vi "Number_Display_Subvi.vi"(6 "Str_x1":refnum<vi>, 7 "Totol Number":i32, 8 "Str_10":refnum<vi>, 9 "Str_x100":refnum<vi>, 10 "Str_x1000":refnum<vi>, 11 "Str_x10000":refnum<vi>) -> ()   [LabVIEW 2013]
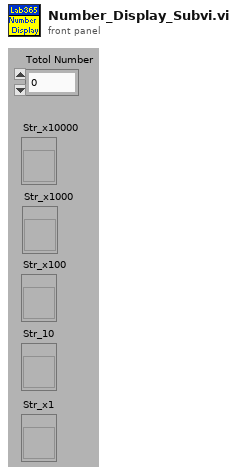
[diagram p1: front panel]
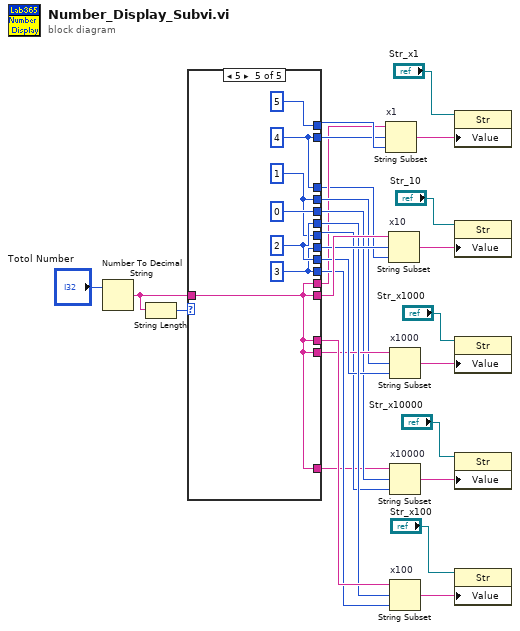
[diagram p0: block diagram]
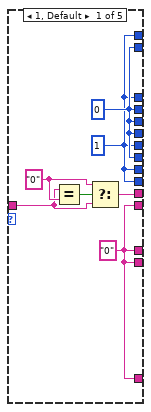
[diagram p2: hidden frame]
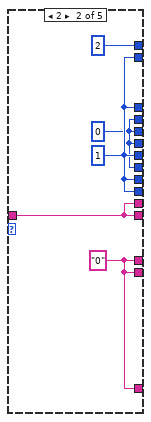
[diagram p3: hidden frame]
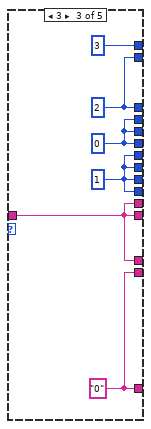
[diagram p4: hidden frame]
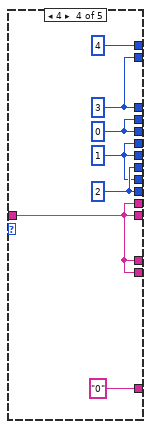
[diagram p5: hidden frame]
diagram:
  n1 = Number To Decimal String(number="Totol Number") -> (decimal integer string=w24:string)  [unwired: 1 out]
  n2 = String Length(string=w24) -> (length=w25:i32)
  n3 = case shown="5" w25 {
    tunnel: w24 -> [w31 w37 w45 w52 w60]
    tunnel: [w32 w37 w45 w52 w60] -> w11
    tunnel: [w30 w38 w41 w47 0 ("长度（剩余）")] -> w14
    tunnel: [w30 w39 w43 w50 w54] -> w16
    tunnel: [w35 w37 w45 w52 w60] -> w23
    tunnel: [w30 w38 w42 w49 w55] -> w22
    tunnel: [w29 w39 w43 w50 w54] -> w9
    tunnel: [w35 w36 w45 w52 w60] -> w21
    tunnel: [w30 w38 w41 w48 w58] -> w20
    tunnel: [w29 w39 w42 w49 w55] -> w19
    tunnel: [w35 w36 w44 w52 w60] -> w15
    tunnel: [w30 w38 w41 w47 w56] -> w13
    tunnel: [w29 w39 w42 w48 w58] -> w18
    tunnel: [w35 w36 w44 "0" w60] -> w10
    tunnel: [w29 w39 w42 w48 w56] -> w12
    tunnel: [w29 2 3 4 ("长度（剩余）") 5 ("长度（剩余）")] -> w17
    frame 1, Default {
      w33 = "0" ("y")
      w35 = "0"
      w29 = 1
      w30 = 0
      n4 = Equal?(x=w31, y=w33) -> (x = y?=w34:bool)
      n5 = Select(t=w33, s=w34, f=w31) -> (s? t:f=w32:string)
    }
    frame 2 {
      w39 = 1 ("长度（剩余）")
      w38 = 0 ("长度（剩余）")
      w36 = "0"
    }
    frame 3 {
      w44 = "0"
      w42 = 1 ("长度（剩余）")
      w43 = 2 ("长度（剩余）")
      w41 = 0 ("长度（剩余）")
    }
    frame 4 {
      w47 = 0 ("偏移量(0)")
      w48 = 1 ("长度（剩余）")
      w49 = 2 ("长度（剩余）")
      w50 = 3 ("长度（剩余）")
    }
    frame 5 {
      w56 = 1 ("长度（剩余）")
      w58 = 2 ("长度（剩余）")
      w55 = 3
      w54 = 4 ("长度（剩余）")
    }
  }
  n6 = String Subset "x1"(string=w11, offset (0)=w16, length (rest)=w17) -> (substring=w27:string)
  n7 = String Subset "x10"(string=w23, offset (0)=w22, length (rest)=w9) -> (substring=w26:string)
  n8 = String Subset "x1000"(string=w15, offset (0)=w13, length (rest)=w18) -> (substring=w6:string)
  n9 = String Subset "x10000"(string=w10, offset (0)=w14, length (rest)=w12) -> (substring=w7:string)
  n10 = String Subset "x100"(string=w21, offset (0)=w20, length (rest)=w19) -> (substring=w8:string)
  n11 = property class="Str"(reference="Str_x1", "Value"=w27) -> ()  [unwired: 1 in, 2 out]
  n12 = property class="Str"(reference="Str_10", "Value"=w26) -> ()  [unwired: 1 in, 2 out]
  n13 = property class="Str"(reference="Str_x1000", "Value"=w6) -> ()  [unwired: 1 in, 2 out]
  n14 = property on="属性节点" class="Str"(reference="Str_x10000", "Value"=w7) -> ()  [unwired: 1 in, 2 out]
  n15 = property class="Str"(reference="Str_x100", "Value"=w8) -> ()  [unwired: 1 in, 2 out]
